vi "AET Clamp ROI subVI.vi"(8 "error in (no error)":errorcluster, 9 "Angle (Pixel)":dbl, 10 "Clamp param":T2, 11 "Edge Information":T3[](array[typedef]) {"Distance (Real-World)" format="%.2f"; "Location (Real-World)"."Y" format="%.2g"; "Location (Real-World)"."X" format="%.2f"; "Noise" format="%.2f"; "Location (Pixel)"."Y" format="%.2g"; "Location (Pixel)"."X" format="%.2f"; "Strength" format="%.2f"; "Distance (Pixel)" format="%.2f"}) -> (0 "error out":errorcluster, 2 "ROI for AET Clamp":T1, 5 "Average X of Contact gap area or center x of contact gap area":sgl)   [LabVIEW 2019, in "Algorithm.lvclass"]
uses:
  FrameworkOverrides/Algorithm.lvclass
  <vilib>/vision/Measure.llb/Edge New.ctl
panel:
  out "Center Y of Contact gap area":sgl
  # "INPUTS"
  # "OUTPUTS"
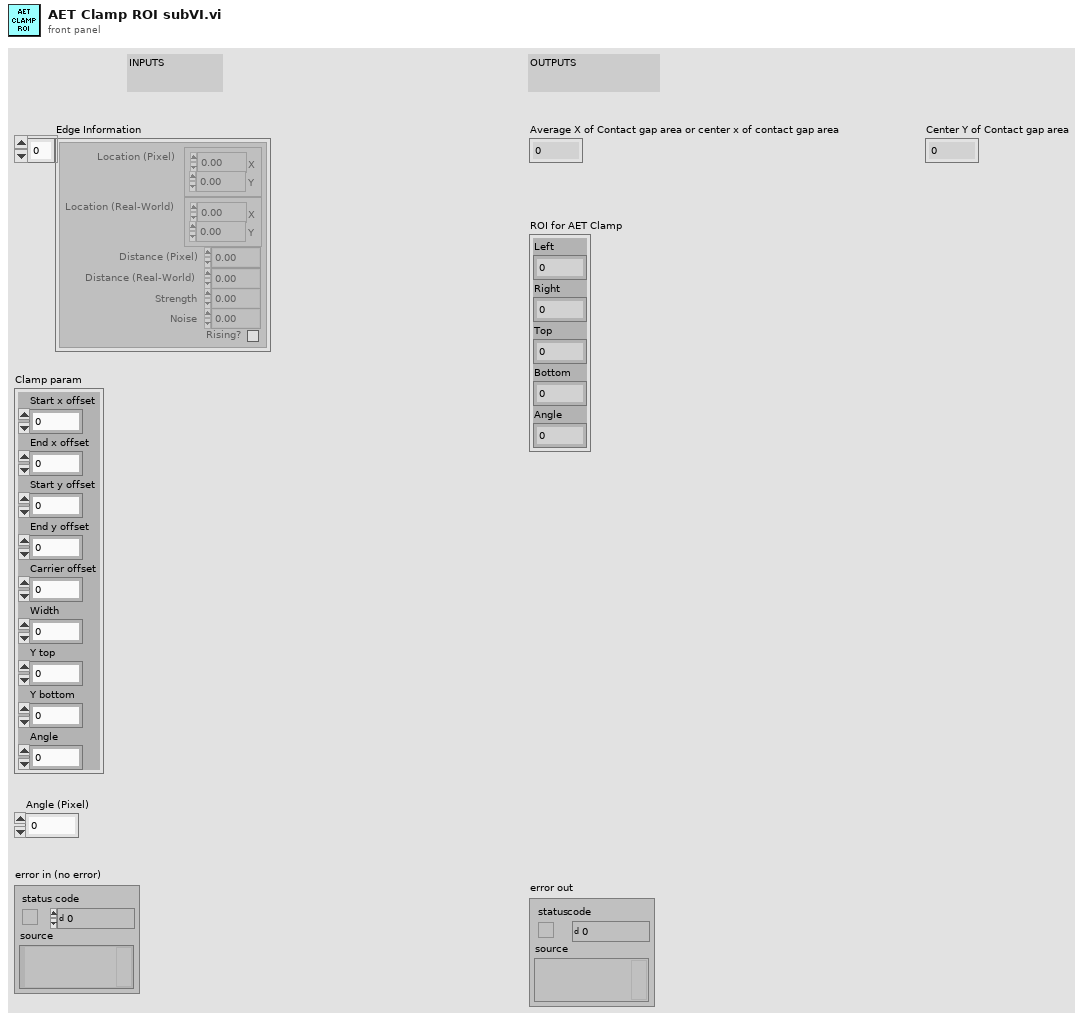
[diagram p1: front panel]
types:
  T1 = cluster{"Left":i32, "Right":i32, "Top ":i32, "Bottom":i32, "Angle":dbl}
  T2 = cluster{"Start x offset":sgl, "End x offset":sgl, "Start y offset":sgl, "End y offset":sgl, "Carrier offset":sgl, "Width":sgl, "Y top":sgl, "Y bottom":sgl, "Angle":sgl}
  T3 = typedef "Edge New.ctl" = cluster{"Location (Pixel)":cluster{"X":sgl, "Y":sgl}, "Location (Real-World)":cluster{"X":sgl, "Y":sgl}, "Distance (Pixel)":dbl, "Distance (Real-World)":dbl, "Strength":dbl, "Noise":dbl, "Rising?":bool}
  T4 = typedef "IMAQ Rectangle" = cluster{"Left":i32, "Top":i32, "Right":i32, "Bottom":i32, "Rotation":dbl}
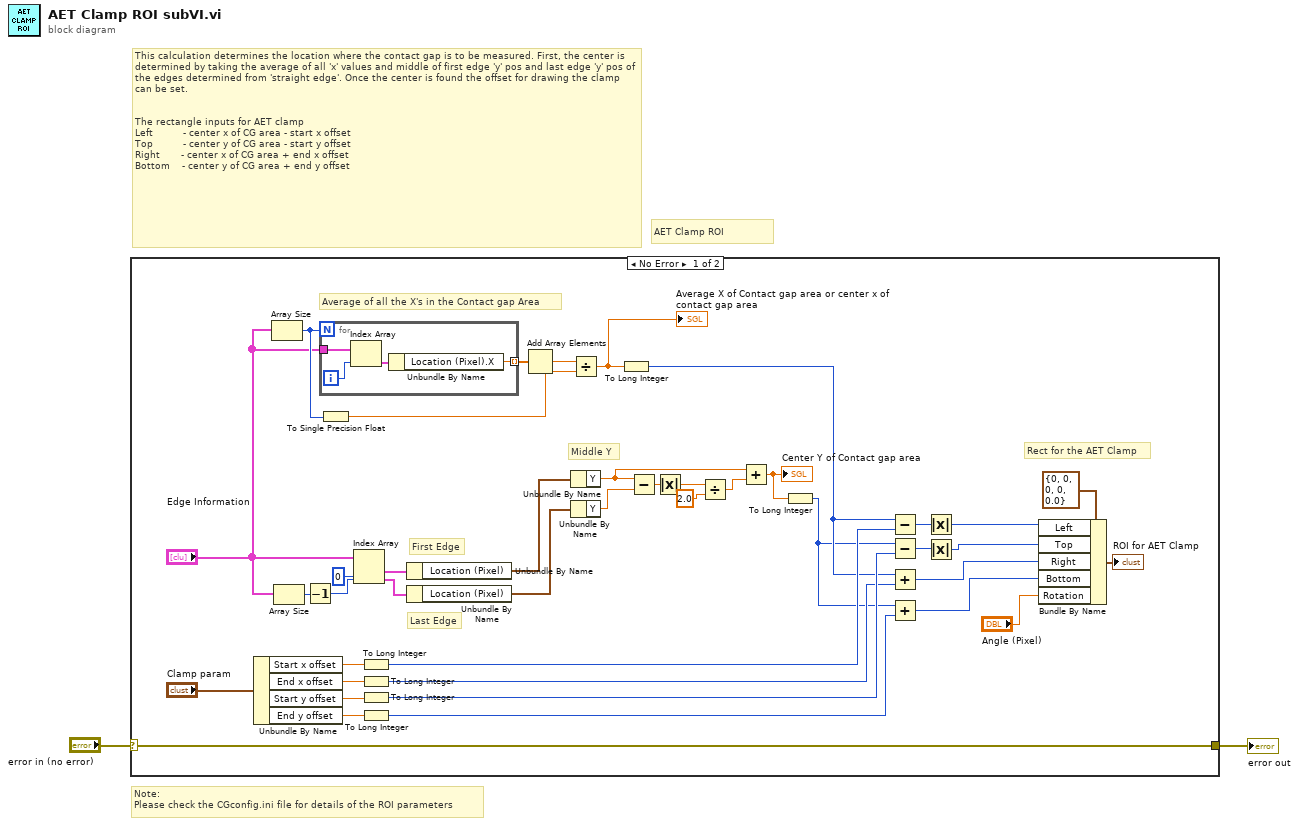
[diagram p0: block diagram]
diagram:
  # "Note:\nPlease check the CGconfig.ini file for details of the ROI parameters"
  # "This calculation determines the location where the contact gap is to be measured. First, the center is determined by taking the average of all 'x' values and middle of first edge 'y' pos and last edge 'y' pos of the edges determined from 'straight edge'. Once the center is found the offset for drawing the clamp can be set.\n\n\nThe rectangle inputs for AET clamp\nLeft          - center x of CG area - start x offset\nTop          - center y of CG area - start y offset \nRight       - center x of CG area + end x offset\nBottom    - center y of CG area + end y offset"
  # "AET Clamp ROI"
  n1 = case shown="No Error" "error in (no error)" {
    selector: "error in (no error)" -> [w23 w48]
    tunnel: [w23 w48] -> w1
    frame No Error {
      # "Average of all the X's in the Contact gap Area"
      # "Rect for the AET Clamp"
      # "Middle Y"
      # "Last Edge"
      # "First Edge"
      n2 = Unbundle By Name("Clamp param") -> ("Start x offset"=w15:sgl, "End x offset"=w7:sgl, "Start y offset"=w20:sgl, "End y offset"=w18:sgl)
      n3 = Array Size(array="Edge Information") -> (size(s)=w27:i32)
      n4 = Array Size(array="Edge Information") -> (size(s)=w42:i32)
      n5 = Decrement(x=w42) -> (x-1=w41:i32)
      n6 = for {
        N: w27 -> [_]
        tunnel: "Edge Information" -> [w47]
        tunnel: [w44] -> w29 mode=indexing
        i -> [w46]
        n7 = Index Array(array=w47, index=w46) -> (element=w45:T3)
        n8 = Unbundle By Name(w45) -> ("Location (Pixel).X"=w44:sgl)
      }
      n9 = To Single Precision Float(number=w27) -> (single precision float=w26:sgl)
      n10 = Index Array(array="Edge Information", index #1=0 ("index"), index #2=w41) -> (element #1=w39:T3, element #2=w43:T3)
      n11 = To Long Integer(number=w15) -> (32bit integer=w14:i32)
      n12 = To Long Integer(number=w7) -> (32bit integer=w6:i32)
      n13 = To Long Integer(number=w20) -> (32bit integer=w19:i32)
      n14 = To Long Integer(number=w18) -> (32bit integer=w17:i32)
      n15 = Unbundle By Name(w39) -> ("Location (Pixel)"=w37:cluster{"X":sgl, "Y":sgl})
      n16 = Unbundle By Name(w43) -> ("Location (Pixel)"=w36:cluster{"X":sgl, "Y":sgl})
      n17 = Add Array Elements(numeric array=w29) -> (sum=w28:sgl)
      n18 = Divide(x=w28, y=w26) -> (x/y=w24:sgl)
      "Average X of Contact gap area or center x of contact gap area" <- w24
      n19 = Unbundle By Name(w37) -> ("Y"=w30:sgl)
      n20 = Unbundle By Name(w36) -> ("Y"=w34:sgl)
      n21 = To Long Integer(number=w24) -> (32bit integer=w8:i32)
      n22 = Subtract(x=w30, y=w34) -> (x-y=w35:sgl)
      n23 = Absolute Value(x=w35) -> (abs(x)=w32:sgl)
      n24 = Divide(x=w32, y=sgl 2.0) -> (x/y=w31:sgl)
      n25 = Add(x=w30, y=w31) -> (x+y=w11:sgl)
      "Center Y of Contact gap area" <- w11
      n26 = To Long Integer(number=w11) -> (32bit integer=w5:i32)
      n27 = Subtract(x=w8, y=w14) -> (x-y=w13:i32)
      n28 = Subtract(x=w5, y=w19) -> (x-y=w10:i32)
      n29 = Add(x=w8, y=w6) -> (x+y=w4:i32)
      n30 = Add(x=w5, y=w17) -> (x+y=w3:i32)
      n31 = Absolute Value(x=w13) -> (abs(x)=w12:i32)
      n32 = Absolute Value(x=w10) -> (abs(x)=w9:i32)
      n33 = Bundle By Name(cluster=T4 {"Left"=0, "Top"=0, "Right"=0, "Bottom"=0, "Rotation"=0.0} ("Rectangle"), "Left"=w12, "Top"=w9, "Right"=w4, "Bottom"=w3, "Rotation"="Angle (Pixel)") -> (→"ROI for AET Clamp":T4)
    }
    frame Error {
    }
  }
  "error out" <- w1
